vi "Launch New Chat Window.vi"(8 "error in (no error)":errorcluster, 11 "Server in":refnum<class "Server.lvclass">) -> (0 "error out":errorcluster, 3 "Server out":refnum<class "Server.lvclass">)   [LabVIEW 2020, in "Server.lvlib" / "Server.lvclass"]
uses:
  Server.lvclass
  C:/Program Files/National Instruments/LabVIEW 2020/vi.lib/ActorFramework/Actor/Actor.lvclass
  Chat Window Model/Chat Window Model/Chat Window Model.lvclass
  Server Messages/Status Update Msg/Status Update Msg.lvclass
  C:/Users/huipeng8/Desktop/SubPanel-Actor-Framework-master/Video 12 - LabVIEW Maps/Chat Window Model/Chat Window Model Messages/Status Updated Msg/Status Updated Msg.lvclass
  Server Messages/Direct Message Recieved Msg/Direct Message Recieved Msg.lvclass
  C:/Users/huipeng8/Desktop/SubPanel-Actor-Framework-master/Video 12 - LabVIEW Maps/Chat Window Model/Chat Window Model Messages/Direct Message Sent Msg/Direct Message Sent Msg.lvclass
  Server Messages/New Reference Recieved Msg/New Reference Recieved Msg.lvclass
  C:/Users/huipeng8/Desktop/SubPanel-Actor-Framework-master/Video 12 - LabVIEW Maps/Chat Window Model/Chat Window Model Messages/New UI Reference Msg/New UI Reference Msg.lvclass
  <vilib>/ActorFramework/Message Enqueuer/Message Enqueuer.lvclass
  Chat Window Model/Chat Window Model/Chat Window Model.lvclass/Chat Window Model.ctl
  <vilib>/ActorFramework/Actor/Actor.lvclass/Actor.ctl
  <vilib>/ActorFramework/Message Enqueuer/Message Enqueuer.lvclass/Message Enqueuer.ctl
  Server.lvclass/Server.ctl
  Server Messages/Enable Controls Msg/Enable Controls Msg.lvclass/Enable Controls Msg.ctl
  Chat Window Model/Chat Window Model Messages/Update Status Log Msg/Update Status Log Msg.lvclass/Update Status Log Msg.ctl
  Chat Window Model/Chat Window Model Messages/Update Online List Msg/Update Online List Msg.lvclass/Update Online List Msg.ctl
  <vilib>/ActorFramework/Message Enqueuer/Init from Existing Queue.vi
  <vilib>/ActorFramework/Message Enqueuer/Enqueue.vi
  Server Messages/Enable Controls Msg/Enable Controls Msg.lvclass
  C:/Program Files/National Instruments/LabVIEW 2020/vi.lib/ActorFramework/Message/Message.lvclass
  Chat Window Model/Chat Window Model Messages/Update Status Log Msg/Update Status Log Msg.lvclass
  Chat Window Model/Chat Window Model Messages/Update Online List Msg/Update Online List Msg.lvclass
  <vilib>/ActorFramework/Message Priority Queue/Priority Enqueue.vi
  <vilib>/ActorFramework/Actor/Actor.lvclass
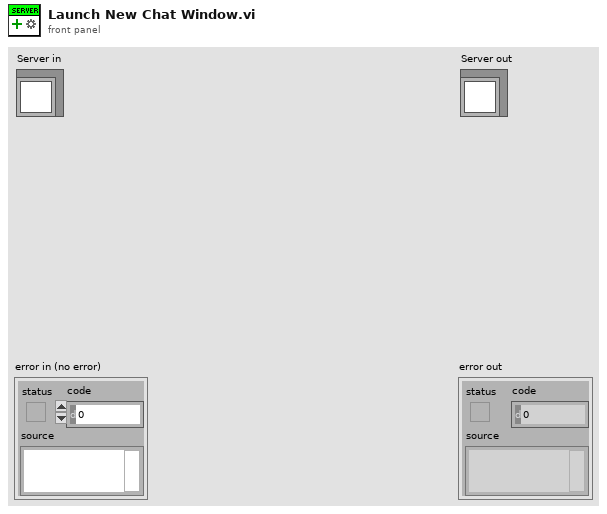
[diagram p1: front panel]
types:
  T1 = cluster{"Enqueuer":refnum<class "Message Enqueuer.lvclass">, "Status":string}
  T2 = enum8{"Enabled", "Disabled", "Disabled and Grayed Out"}
  T3 = map{string, cluster{"Enqueuer":refnum<class "Message Enqueuer.lvclass">, "Status":string}}
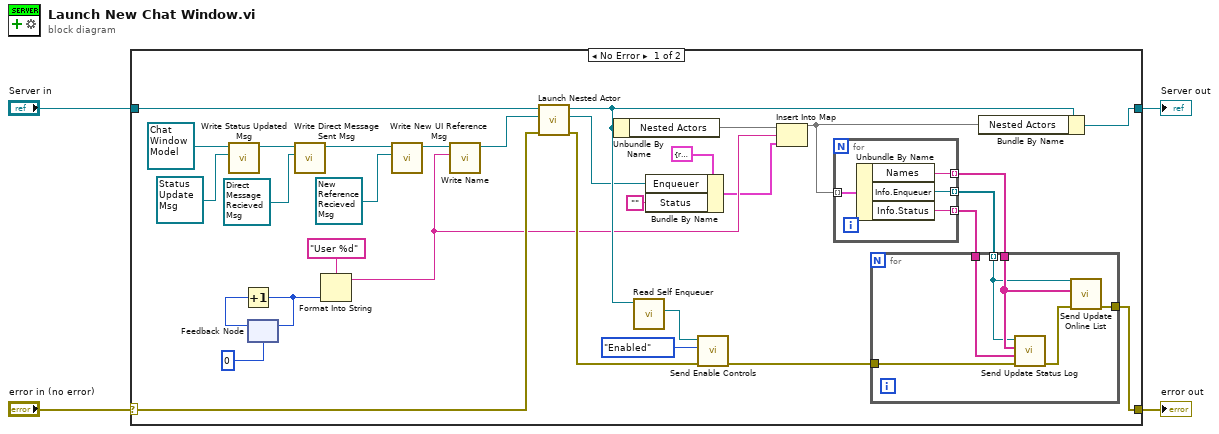
[diagram p0: block diagram]
diagram:
  n1 = case shown="No Error" "error in (no error)" {
    selector: "error in (no error)" -> [w34 w47]
    tunnel: [w23 w47] -> w3
    tunnel: [w24 w46] -> w1
    tunnel: "Server in" -> [w35 w46]
    frame No Error {
      n2 = call "Write Status Updated Msg.vi"("Chat Window Model.lvlib:Status Updated Msg.lvclass"=refnum<class "Status Update Msg.lvclass"> refnum ("Server.lvlib:Status Update Msg.lvclass"), "Chat Window Model in"=refnum<class "Chat Window Model.lvclass"> refnum ("Chat Window Model.lvlib:Chat Window Model.lvclass")) -> ("Chat Window Model out"=w26:refnum<class "Chat Window Model.lvclass">)  [unwired: 9 in]
      n3 = feedback #1(0) -> (w31:i32)
      n4 = Increment(x=w31) -> (x+1=w29:i32)
      n5 = feedback-in #1(w29) -> ()
      n6 = call "Write Direct Message Sent Msg.vi"("Chat Window Model.lvlib:Direct Message Sent Msg.lvclass"=refnum<class "Direct Message Recieved Msg.lvclass"> refnum ("Server.lvlib:Direct Message Recieved Msg.lvclass"), "Chat Window Model in"=w26) -> ("Chat Window Model out"=w17:refnum<class "Chat Window Model.lvclass">)  [unwired: 9 in]
      n7 = Format Into String(format string="User %d", w29) -> (resulting string=w13:string)  [unwired: 2 in, 1 out]
      n8 = call "Write New UI Reference Msg.vi"("Chat Window Model.lvlib:New UI Reference Msg.lvclass"=refnum<class "New Reference Recieved Msg.lvclass"> refnum ("Server.lvlib:New Reference Recieved Msg.lvclass"), "Chat Window Model in"=w17) -> ("Chat Window Model out"=w16:refnum<class "Chat Window Model.lvclass">)  [unwired: 9 in]
      n9 = call "Write Name.vi"("Name"=w13, "Chat Window Model in"=w16) -> ("Chat Window Model out"=w33:refnum<class "Chat Window Model.lvclass">)  [unwired: 8 in, 1 out]
      n10 = call <vilib>:"Launch Nested Actor.vi"("error in (no error)"=w34, "Nested Actor"=w33, "Caller Actor in"=w35) -> ("error out"=w21:errorcluster, "Nested Actor's Enqueuer"=w11:refnum<class "Message Enqueuer.lvclass">, "Caller Actor out"=w20:refnum<class "Server.lvclass">)  [unwired: 6 in]
      n11 = Unbundle By Name(w20) -> ("Nested Actors"=w14:T3)
      n12 = call <vilib>:"Read Self Enqueuer.vi"("Actor"=w20) -> ("Self Enqueuer"=w19:refnum<class "Message Enqueuer.lvclass">)  [unwired: 10 in]
      n13 = Bundle By Name(cluster=T1 {"Enqueuer"=refnum, "Status"=""} ("value"), "Enqueuer"=w11, "Status"="") -> (w9:T1)
      n14 = call "Send Enable Controls.vi"("error in (no error)"=w21, "Disabled"=T2."Enabled", "Message Enqueuer"=w19) -> ("error out"=w22:errorcluster)  [unwired: 7 in, 1 out]
      n15 = Insert Into Map(map in=w14, key=w13, value=w9) -> (map out=w8:T3)  [unwired: 2 out]
      n16 = for {
        tunnel: [w38] -> w7 mode=indexing
        tunnel: w8 -> [w39] mode=indexing
        tunnel: [w37] -> w6 mode=indexing
        tunnel: [w36] -> w5 mode=indexing
        n17 = Unbundle By Name(w39) -> ("Names"=w38:string, "Info.Enqueuer"=w37:refnum<class "Message Enqueuer.lvclass">, "Info.Status"=w36:string)
      }
      n18 = for {
        tunnel: [w44] -> w23
        tunnel: w22 -> [w43]
        tunnel: w7 -> [w42]
        tunnel: w6 -> [w41] mode=indexing
        tunnel: w5 -> [w40]
        n19 = call "Send Update Status Log.vi"("error in (no error)"=w43, "Status List"=w40, "Names"=w42, "Message Enqueuer"=w41) -> ("error out"=w45:errorcluster)  [unwired: 6 in, 1 out]
        n20 = call "Send Update Online List.vi"("error in (no error)"=w45, "Online Users"=w42, "Message Enqueuer"=w41) -> ("error out"=w44:errorcluster)  [unwired: 7 in, 1 out]
      }
      n21 = Bundle By Name(cluster=w20, "Nested Actors"=w8) -> (w24:refnum<class "Server.lvclass">)
    }
    frame Error {
    }
  }
  "error out" <- w3
  "Server out" <- w1
